vi "PH_Beckhoff_PP_Control.handle PP Conductivity.vi"(0 "i ref in":refnum<vi>, 1 "changed DE Values":i32[](array[numeric]), 3 "Current Digital Inputs":T1, 5 "error in":errorcluster) -> (14 "i ref out":refnum<vi>, 19 "error out":errorcluster)   [LabVIEW 2014, in "PH_Beckhoff_PP_Control.lvlib"]
doc: "This VI handles all information related to the PP conductivity measurement (KOBO LF). If it changed, it publishes the current status and sets the related GUI element."
uses:
  PH_Beckhoff_PP_Control.lvlib
  PH_Beckhoff/PH_Beckhoff.Digital Inputs.ctl
  PH_Basics/PH_StatusHandler/PH_StatusHandler.Status.ctl
  PH_Basics/PH_StatusHandler/PH_StatusHandler.lvlib
  PH_Basics/PH_Common/PH_Common.lvlib
  PH_Beckhoff/PH_Beckhoff.lvlib
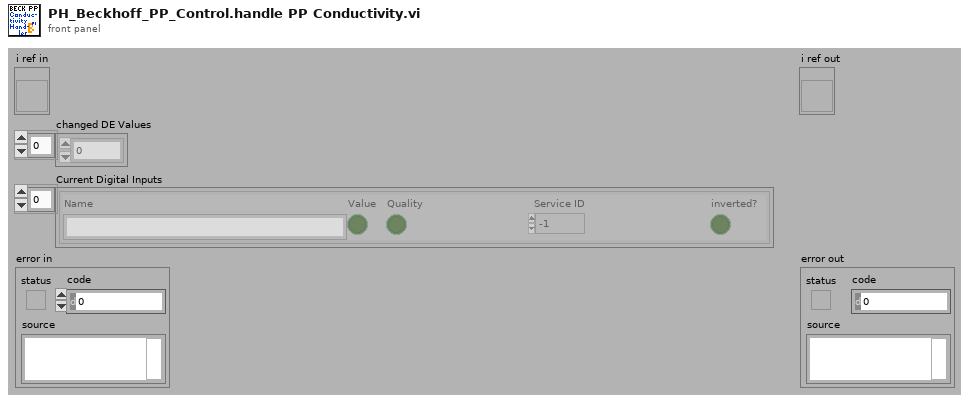
[diagram p1: front panel]
types:
  T1 = typedef "PH_Beckhoff.lvlib/PH_Beckhoff.Digital Inputs.ctl" = cluster{"Name":string, "Value":bool, "Quality":bool, "Service ID":i32, "inverted?":bool}[]
  T2 = typedef "PH_Beckhoff_PP_Control.lvlib/PH_Beckhoff_PP_Control.i attribute.ctl" = cluster{"PP Conductivity Control":cluster{"PSDB":cluster{"Status Service ID":i32, "Instance ID":i32, "Data Status":T3, "Ref Status":refnum<vi>, "Error Code":i32}, "Status":cluster{"GUI Ref":refnum<vi>, "Status Service ID":i32, "Status":T4}, "DIs":cluster{"Device on":cluster{"GUI Ref":refnum<vi>, "# in Data":i32}, "Conductivity ok":cluster{"GUI Ref":refnum<vi>, "# in Data":i32}, "Temperature ok":cluster{"GUI Ref":refnum<vi>, "# in Data":i32}, "Alarm":cluster{"GUI Ref":refnum<vi>, "# in Data":i32}}, "PSDB Thread":cluster{"Ref":refnum<vi>, "Q-Ref":refnum<queue>}}, "PP Mercury Control":cluster{"PSDB":cluster{"Status Service ID":i32, "Instance ID":i32, "Data Status":T3, "Ref Status":refnum<vi>, "Error Code":i32}, "Status":cluster{"GUI Ref":refnum<vi>, "Status Service ID":i32, "Status":T4}, "on since:":cluster{"GUI Ref":refnum<vi>, "Service ID":i32, "Time":string}, "DIs":cluster{"Device on":cluster{"GUI Ref":refnum<vi>, "# in Data":i32}, "Alarm":cluster{"GUI Ref":refnum<vi>, "# in Data":i32}}, "AIs":cluster{"Concentration":cluster{"GUI Ref":refnum<vi>, "# in Data":i32}}, "PSDB Thread":cluster{"Ref":refnum<vi>, "Q-Ref":refnum<queue>}}, "PSDB":cluster{"Shot #":i32, "Subsystem":T5}, "PSDB Credentials":T6}
  T3 = typedef "PH_PSDBWriter.lvlib/PH_PSDBWriter.Data Status.ctl" = i16
  T4 = typedef "PH_StatusHandler.lvlib/PH_StatusHandler.Status.ctl" = i16
  T5 = typedef "PH_PSDBWriter.lvlib/PH_PSDBWriter.PHELIX-Subsystems.ctl" = i32
  T6 = typedef "PH_Common.lvlib/PH_Connection.PSDB Credentials.ctl" = cluster{"PW":string, "ID":string, "DS":string}
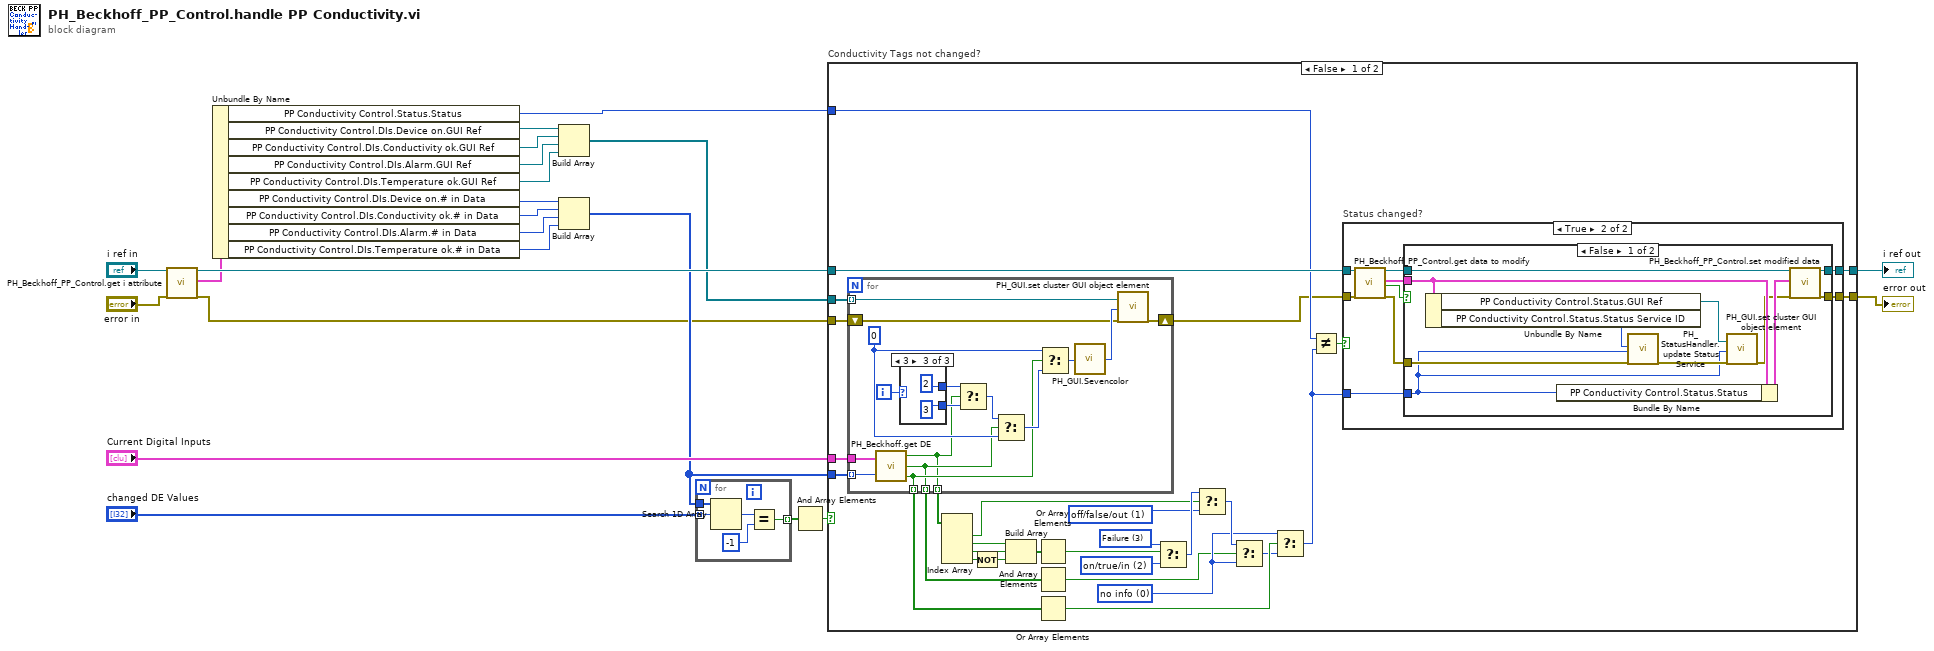
[diagram p0: block diagram]
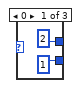
[diagram p2: hidden frame]
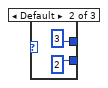
[diagram p3: hidden frame]
diagram:
  n1 = call "PH_Beckhoff_PP_Control.get i attribute.vi"("i ref in"="i ref in", "error in (no error)"="error in") -> ("i ref out"=w19:refnum<vi>, "i attribute"=w18:T2, "error out"=w2:errorcluster)  [unwired: 15 in]
  n2 = Unbundle By Name(w18) -> ("PP Conductivity Control.Status.Status"=w17:T4, "PP Conductivity Control.DIs.Device on.GUI Ref"=w15:refnum<vi>, "PP Conductivity Control.DIs.Conductivity ok.GUI Ref"=w14:refnum<vi>, "PP Conductivity Control.DIs.Alarm.GUI Ref"=w13:refnum<vi>, "PP Conductivity Control.DIs.Temperature ok.GUI Ref"=w12:refnum<vi>, "PP Conductivity Control.DIs.Device on.# in Data"=w11:i32, "PP Conductivity Control.DIs.Conductivity ok.# in Data"=w10:i32, "PP Conductivity Control.DIs.Alarm.# in Data"=w9:i32, "PP Conductivity Control.DIs.Temperature ok.# in Data"=w8:i32)
  n3 = Build Array(w15, w14, w13, w12) -> (w5:refnum<vi>[])
  n4 = Build Array(w11, w10, w9, w8) -> (w3:i32[])
  n5 = for {
    tunnel: w3 -> [w27]
    tunnel: "changed DE Values" -> [w26] mode=indexing
    tunnel: [w25] -> w6 mode=indexing
    n6 = Search 1D Array(1D array=w27, element=w26) -> (index of element=w24:i32)  [unwired: 1 in]
    n7 = Equal?(x=w24, y=-1) -> (x = y?=w25:bool)
  }
  n8 = And Array Elements(Boolean array=w6) -> (logical AND=w1:bool)
  n9 = case "Conductivity Tags not changed?" shown="False" w1 {
    tunnel: [w54 w105] -> w22
    tunnel: w19 -> [w38 w105]
    tunnel: w17 -> [w37 _]
    tunnel: [w36 w104] -> w16
    tunnel: w5 -> [w35 _]
    tunnel: "Current Digital Inputs" -> [w34 _]
    tunnel: w3 -> [w33 _]
    tunnel: w2 -> [w30 w104]
    frame False {
      w52 = T4 3 items=["no info", "off/false/out", "on/true/in", "Failure", "Alarm", "Status 1", "Status 2", "Status 3"] ("Device Status")
      w51 = T4 2 items=["no info", "off/false/out", "on/true/in", "Failure", "Alarm", "Status 1", "Status 2", "Status 3"] ("Device Status")
      w44 = T4 1 items=["no info", "off/false/out", "on/true/in", "Failure", "Alarm", "Status 1", "Status 2", "Status 3"] ("Device Status")
      w40 = T4 0 items=["no info", "off/false/out", "on/true/in", "Failure", "Alarm", "Status 1", "Status 2", "Status 3"] ("Device Status")
      n10 = for {
        shift-right: [w65] -> w29
        shift-left: w30 -> [w64]
        tunnel: w35 -> [w63] mode=indexing
        tunnel: [w58] -> w28 mode=indexing
        tunnel: [w59] -> w32 mode=indexing
        tunnel: [w60] -> w31 mode=indexing
        tunnel: w34 -> [w62]
        tunnel: w33 -> [w61] mode=indexing
        i -> [w67]
        w72 = 0 ("State")
        n11 = call "PH_Beckhoff.get DE.vi"("Digital Values"=w62, "index of element"=w61) -> ("Value"=w58:bool, "Quality"=w59:bool, "Tag not found"=w60:bool)
        n12 = case shown="3" w67 {
          tunnel: [2 ("State") 3 ("State") 2 ("State")] -> w69
          tunnel: [1 ("State") 2 ("State") 3 ("State")] -> w68
          frame 0 {
          }
          frame Default {
          }
          frame 3 {
          }
        }
        n13 = Select(t=w69, s=w58, f=w68) -> (s? t:f=w70:i32)
        n14 = Select(t=w70, s=w59, f=w72) -> (s? t:f=w71:i32)
        n15 = Select(t=w72, s=w60, f=w71) -> (s? t:f=w73:i32)
        n16 = call "PH_GUI.Sevencolor.vi"("State"=w73) -> ("Color Box"=w66:u32)
        n17 = call "PH_GUI.set cluster GUI object element.vi"("Ctl Refnum"=w63, "Value"=w66, "error in"=w64) -> ("error out"=w65:errorcluster)  [unwired: 16 in]
      }
      n18 = Index Array(array=w28) -> (element #1=w42:bool, element #2=w45:bool, element #3=w46:bool, element #4=w47:bool)  [unwired: 4 in]
      n19 = Not(x=w47) -> (.not. x?=w48:bool)
      n20 = Build Array(w45, w46, w48) -> (w49:bool[])
      n21 = Or Array Elements(Boolean array=w49) -> (logical OR=w50:bool)
      n22 = And Array Elements(Boolean array=w32) -> (logical AND=w39:bool)
      n23 = Or Array Elements(Boolean array=w31) -> (logical OR=w57:bool)
      n24 = Select(t=w52, s=w50, f=w51) -> (s? t:f=w53:T4)
      n25 = Select(t=w53, s=w42, f=w44) -> (s? t:f=w43:T4)
      n26 = Select(t=w43, s=w39, f=w40) -> (s? t:f=w41:T4)
      n27 = Select(t=w40, s=w57, f=w41) -> (s? t:f=w56:T4)
      n28 = Not Equal?(x=w37, y=w56) -> (x != y?=w55:bool)
      n29 = case "Status changed?" shown="True" w55 {
        tunnel: w29 -> [w80 w90]
        tunnel: [w80 w88] -> w36
        tunnel: w38 -> [w81 w87]
        tunnel: [w81 w85] -> w54
        tunnel: w56 -> [_ w82]
        frame False {
        }
        frame True {
          n30 = call "PH_Beckhoff_PP_Control.get data to modify.vi"("i ref in"=w87, "error in (no error)"=w90) -> ("i ref out"=w86:refnum<vi>, "i attribute"=w83:T2, "timed out"=w84:bool, "error out"=w89:errorcluster)  [unwired: 14 in]
          n31 = case shown="False" w84 {
            tunnel: w89 -> [w97 w102]
            tunnel: [w101 w102] -> w88
            tunnel: w86 -> [w100 w103]
            tunnel: [w99 w103] -> w85
            tunnel: w83 -> [w95 _]
            tunnel: w82 -> [w91 _]
            frame False {
              n32 = Unbundle By Name(w95) -> ("PP Conductivity Control.Status.GUI Ref"=w92:refnum<vi>, "PP Conductivity Control.Status.Status Service ID"=w94:i32)
              n33 = Bundle By Name(cluster=w95, "PP Conductivity Control.Status.Status"=w91) -> (w98:T2)
              n34 = call "PH_StatusHandler.update Status Service.vi"("Service ID"=w94, "Status"=w91, "error in (no error)"=w97) -> ("error out"=w96:errorcluster)  [unwired: 16 in]
              n35 = call "PH_GUI.set cluster GUI object element.vi"("Ctl Refnum"=w92, "Value"=w91, "error in"=w96) -> ("error out"=w93:errorcluster)  [unwired: 16 in]
              n36 = call "PH_Beckhoff_PP_Control.set modified data.vi"("i ref in"=w100, "i attribute"=w98, "error in (no error)"=w93) -> ("i ref out"=w99:refnum<vi>, "error out"=w101:errorcluster)  [unwired: 15 in]
            }
            frame True {
            }
          }
        }
      }
    }
    frame True {
    }
  }
  "error out" <- w16
  "i ref out" <- w22
